vi "gfitsio-delete-current-hdu.vi"(8 "error in (no error)":errorcluster, 11 "gfits refnum":T1) -> (0 "error out":errorcluster, 3 "dup gfits refnum":T1)   [LabVIEW 2019, in "gfitsio.lvlib"]
doc: "Delete the current HDU (CHDU) in the FITS file. Any following HDUs will be shifted forward in the file, to fill in the gap created by the deleted HDU. In the case of deleting the primary array (the first HDU in the file) then the current primary array will be replace by a null primary array containing the minimum set of required keywords and no data. If there are more extensions in the file following the one that is deleted, then the the CHDU will be redefined to point to the following extension. If there are no following extensions then the CHDU will be redefined to point to the previous HDU."
uses:
  gfitsio.lvlib
  gfitsio-refnum.ctl
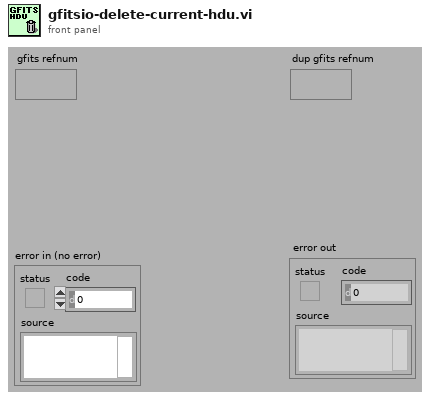
[diagram p1: front panel]
types:
  T1 = typedef "gfitsio.lvlib/gfitsio-refnum.ctl" = refnum<k1>
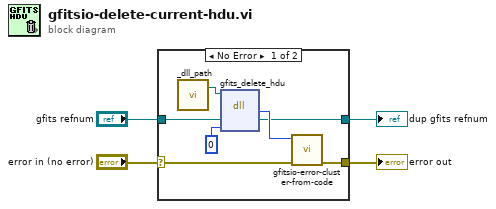
[diagram p0: block diagram]
diagram:
  n1 = case shown="No Error" "error in (no error)" {
    selector: "error in (no error)" -> [w9 w13]
    tunnel: [w11 w13] -> w4
    tunnel: "gfits refnum" -> [w7 w12]
    tunnel: [w8 w12] -> w2
    frame No Error {
      n2 = call "_dll_path.vi"() -> ("Path"=w5:path)  [unwired: 1 in]
      n3 = dll-call lib="?" fn="gfits_delete_hdu"(path in=w5, "refnum"=w7, "tbltype"=0) -> ("return type"=w10:i32, "refnum"=w8:T1)  [unwired: 2 in, 3 out]
      n4 = call "gfitsio-error-cluster-from-code.vi"("error in (no error)"=w9, "error code"=w10) -> ("error out"=w11:errorcluster)  [unwired: 9 out]
    }
    frame Error {
    }
  }
  "error out" <- w4
  "dup gfits refnum" <- w2
